vi "Bounce Window_User Accounts_Table.vi"(7 "User Accounts_Action":T5, 9 "User Account Data":T1={"帳號 :"="", "權限等級："=enum."開發人員", "建立時間："="", "修改時間："="", "到期時間："="", "狀態："=enum."可使用", "期限："=enum."一天", "密碼："=""}, 10 "Row":i32, 11 "User Accounts Table":refnum<vi>) -> ()   [LabVIEW 2015]
uses:
  <vilib>/Utility/miscctls.llb/LVRowAndColumnTypeDef.ctl
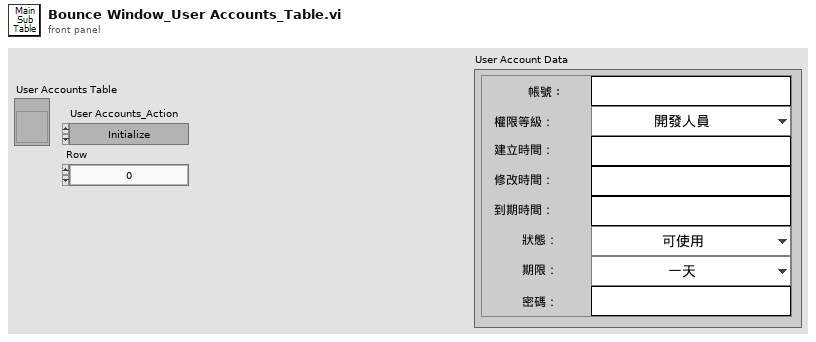
[diagram p1: front panel]
types:
  T1 = typedef "Control_User account_Data.ctl" = cluster{"帳號 :":string, "權限等級：":T2, "建立時間：":string, "修改時間：":string, "到期時間：":string, "狀態：":T3, "期限：":T4, "密碼：":string}
  T2 = typedef "Control_User account_Permissions.ctl" = enum16{"開發人員", "管理者", "工程師", "作業員"}
  T3 = typedef "Control_User Accounts_Status.ctl" = enum16{"可使用", "不可使用"}
  T4 = typedef "Control_User account_Date.ctl" = enum16{"零天", "一天", "七天", "一個月", "一年", "三年"}
  T5 = typedef "Control_Bounce Window_User Accounts_Table Action" = enum16{"Initialize", "Set Data", "Delete Data", "Replace Data", "Close"}
  T6 = typedef "LVRowAndColumnTypeDef.ctl" = cluster{"Row":i32, "Column":i32}
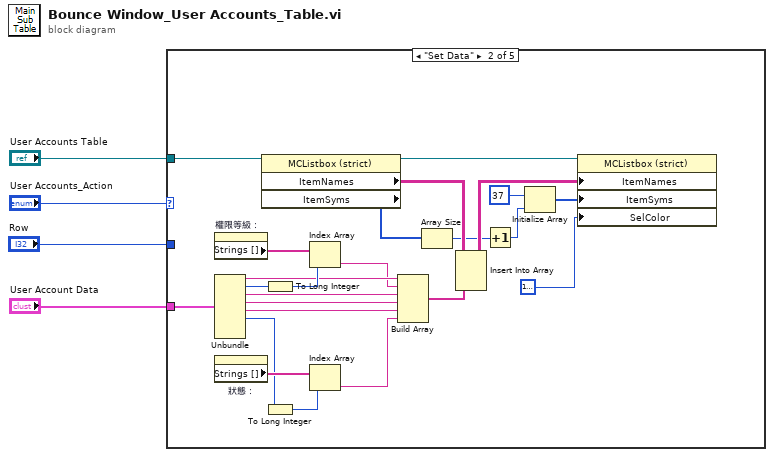
[diagram p0: block diagram]
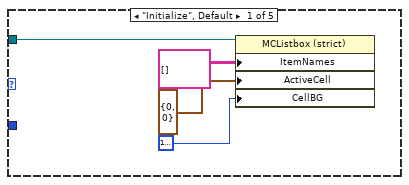
[diagram p2: hidden frame]
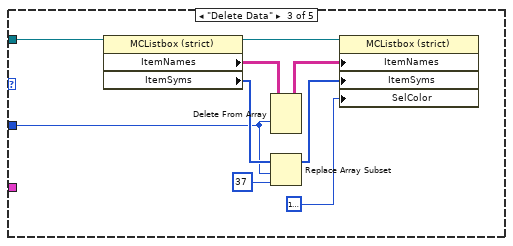
[diagram p3: hidden frame]
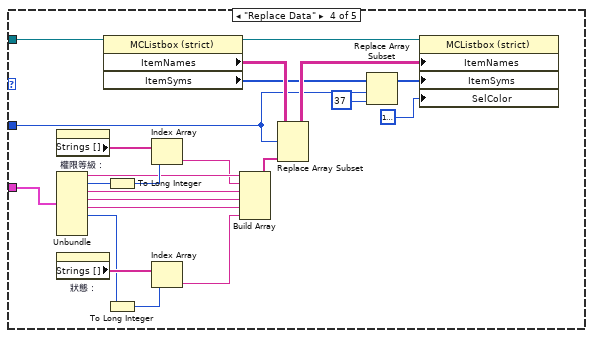
[diagram p4: hidden frame]
diagram:
  n1 = case shown="\"Set Data\"" "User Accounts_Action" {
    tunnel: "User Accounts Table" -> [w8 w32 w38 w47 _]
    tunnel: "User Account Data" -> [_ w14 _ w46 _]
    tunnel: "Row" -> [_ _ w33 w43 _]
    frame "Initialize", Default {
      n2 = property class="MCListbox (strict)"(reference=w8, "ItemNames"=string[][] [] ("Item Names"), "ActiveCell"=T6 {"Row"=0, "Column"=0} ("Active Cell:Active Cell"), "CellBG"=u32 16777225 ("Color Box")) -> ()  [unwired: 1 in, 2 out]
    }
    frame "Set Data" {
      n3 = property on="權限等級：" class="Enum (strict)"() -> ("Strings []"=w30:string[])  [unwired: 2 in, 2 out]
      n4 = Unbundle(w14) -> ("帳號 :"=w24:string, "權限等級："=w29:T2, "建立時間："=w22:string, "修改時間："=w21:string, "到期時間："=w20:string, "狀態："=w25:T3)  [unwired: 2 out]
      n5 = property on="狀態：" class="Enum (strict)"() -> ("Strings []"=w26:string[])  [unwired: 2 in, 2 out]
      n6 = property class="MCListbox (strict)"(reference=w32) -> (reference out=w31:refnum<vi>, "ItemNames"=w13:string[][], "ItemSyms"=w12:i32[])  [unwired: 1 in, 1 out]
      n7 = To Long Integer(number=w29) -> (32bit integer=w28:i32)
      n8 = To Long Integer(number=w25) -> (32bit integer=w27:i32)
      n9 = Index Array(array=w30, index=w28) -> (element=w23:string)
      n10 = Index Array(array=w26, index=w27) -> (element=w19:string)
      n11 = Build Array(w24, w23, w22, w21, w20, w19) -> (w18:string[])
      n12 = Array Size(array=w12) -> (size(s)=w10:i32)
      n13 = Insert Into Array(array=w13, new element=w18) -> (w15:string[][])  [unwired: 2 in]
      n14 = Increment(x=w10) -> (x+1=w11:i32)
      n15 = Initialize Array(37 ("new element/subarray"), w11) -> (w16:i32[])
      n16 = property class="MCListbox (strict)"(reference=w31, "ItemNames"=w15, "ItemSyms"=w16, "SelColor"=u32 16777225 ("Color Box")) -> ()  [unwired: 1 in, 2 out]
    }
    frame "Delete Data" {
      n17 = property class="MCListbox (strict)"(reference=w38) -> (reference out=w41:refnum<vi>, "ItemNames"=w40:string[][], "ItemSyms"=w37:i32[])  [unwired: 1 in, 1 out]
      n18 = Delete From Array(array=w40, index (row)=w33) -> (array with subset deleted=w39:string[][])  [unwired: 2 in, 1 out]
      n19 = Replace Array Subset(array=w37, new element=37 ("new element/subarray"), index=w33) -> (w36:i32[])
      n20 = property class="MCListbox (strict)"(reference=w41, "ItemNames"=w39, "ItemSyms"=w36, "SelColor"=u32 16777225 ("Color Box")) -> ()  [unwired: 1 in, 2 out]
    }
    frame "Replace Data" {
      n21 = property on="權限等級：" class="Enum (strict)"() -> ("Strings []"=w62:string[])  [unwired: 2 in, 2 out]
      n22 = Unbundle(w46) -> ("帳號 :"=w56:string, "權限等級："=w61:T2, "建立時間："=w54:string, "修改時間："=w53:string, "到期時間："=w52:string, "狀態："=w57:T3)  [unwired: 2 out]
      n23 = property on="狀態：" class="Enum (strict)"() -> ("Strings []"=w58:string[])  [unwired: 2 in, 2 out]
      n24 = property class="MCListbox (strict)"(reference=w47) -> (reference out=w64:refnum<vi>, "ItemNames"=w63:string[][], "ItemSyms"=w49:i32[])  [unwired: 1 in, 1 out]
      n25 = To Long Integer(number=w61) -> (32bit integer=w60:i32)
      n26 = To Long Integer(number=w57) -> (32bit integer=w59:i32)
      n27 = Index Array(array=w62, index=w60) -> (element=w55:string)
      n28 = Index Array(array=w58, index=w59) -> (element=w51:string)
      n29 = Build Array(w56, w55, w54, w53, w52, w51) -> (w44:string[])
      n30 = Replace Array Subset(array=w63, new element=w44, index (row)=w43) -> (w50:string[][])  [unwired: 1 in]
      n31 = Replace Array Subset(array=w49, new element=37 ("new element/subarray"), index=w43) -> (w48:i32[])
      n32 = property class="MCListbox (strict)"(reference=w64, "ItemNames"=w50, "ItemSyms"=w48, "SelColor"=u32 16777225 ("Color Box")) -> ()  [unwired: 1 in, 2 out]
    }
    frame "Close" {
    }
  }
